vi "Read Connection.vi"(8 "error in (no error)":errorcluster, 11 "MQTT Client in":refnum<class "MQTT Client.lvclass">) -> (0 "error out":errorcluster, 2 "Connection Config":T1, 3 "MQTT Client out":refnum<class "MQTT Client.lvclass">)   [LabVIEW 2020, in "MQTT Client.lvclass"]
uses:
  MQTT Client.lvclass
  mqttTypedef/ConnectionConfig.ctl
  MQTT Client.lvclass/MQTT Client.ctl
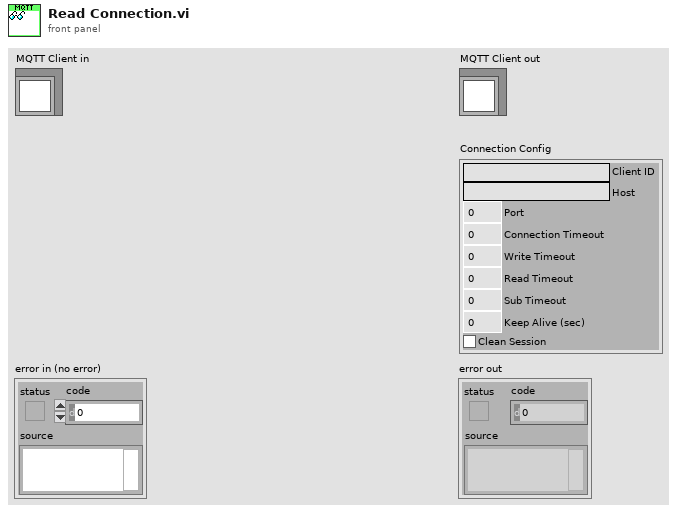
[diagram p1: front panel]
types:
  T1 = typedef "MQTT Client.lvclass/ConnectionConfig.ctl" = cluster{"Client ID":string, "Host":string, "Port":u16, "Connection Timeout":i32, "Write Timeout":i32, "Read Timeout":i32, "Sub Timeout":i32, "Keep Alive (sec)":u16, "Clean Session":bool}
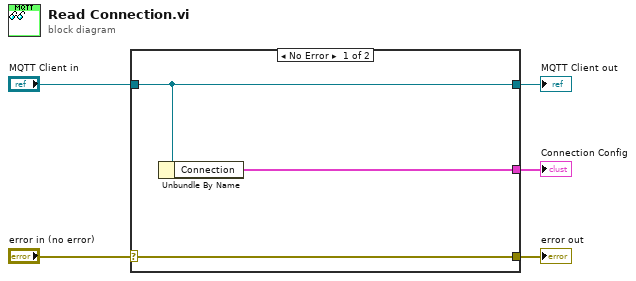
[diagram p0: block diagram]
diagram:
  n1 = case shown="No Error" "error in (no error)" {
    selector: "error in (no error)" -> [w8 w9]
    tunnel: [w8 w9] -> w4
    tunnel: [w7 w10] -> w2
    tunnel: "MQTT Client in" -> [w7 w10]
    tunnel: [w6 _] -> w1
    frame No Error {
      n2 = Unbundle By Name(w7) -> ("Connection"=w6:T1)
    }
    frame Error {
    }
  }
  "error out" <- w4
  "MQTT Client out" <- w2
  "Connection Config" <- w1
